vi "test_system_state-machine.vi"() -> ()   [LabVIEW 2019]
uses:
  Ctrl/main_system.ctl
panel:
  in  "정지":bool
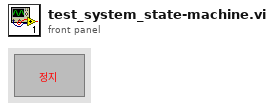
[diagram p1: front panel]
types:
  T1 = typedef "main_system.ctl" = enum16{"init state", "start point check", "end point check", "start angle check", "stop", "wait", "waypoint check"}
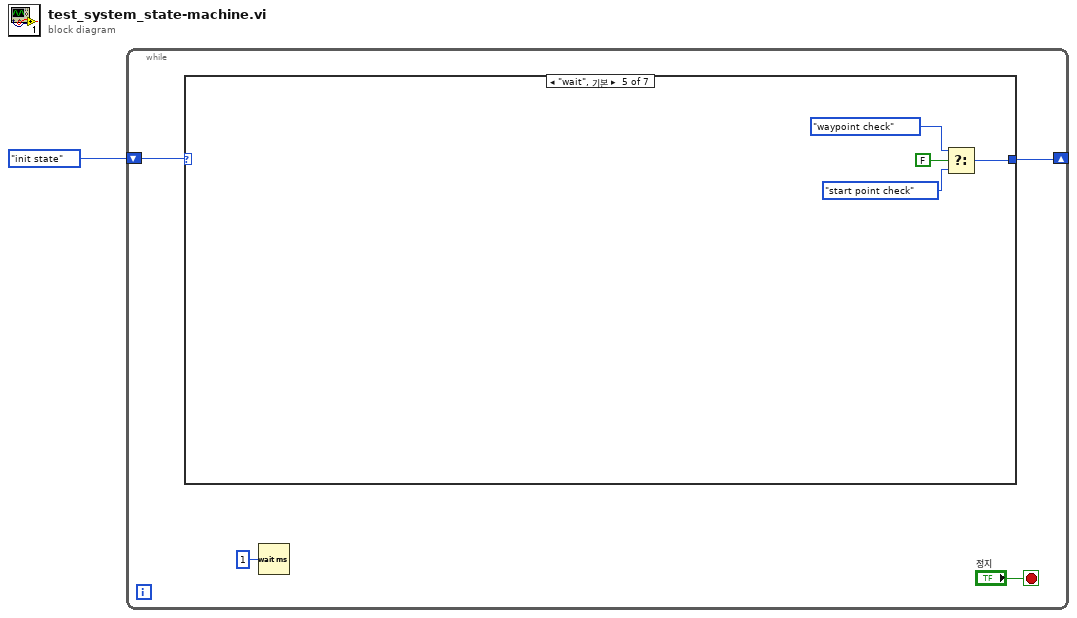
[diagram p0: block diagram]
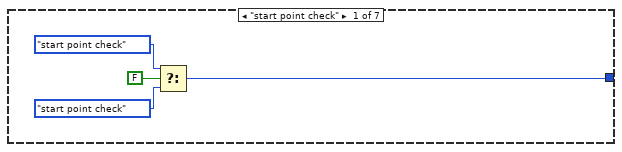
[diagram p2: hidden frame]
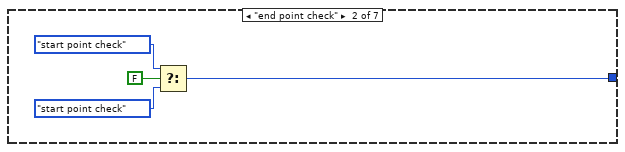
[diagram p3: hidden frame]
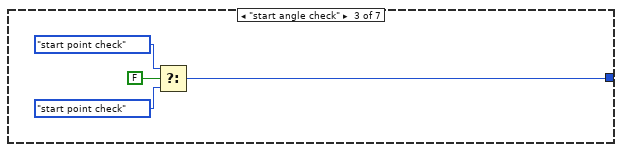
[diagram p4: hidden frame]
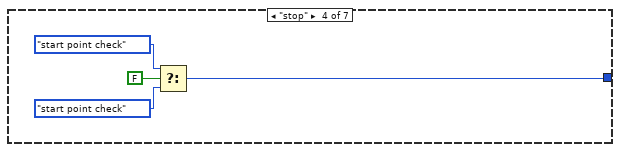
[diagram p5: hidden frame]
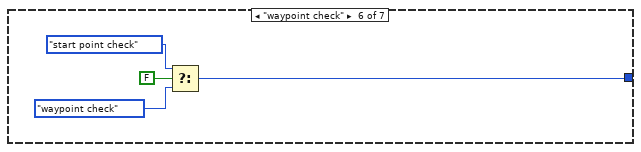
[diagram p6: hidden frame]
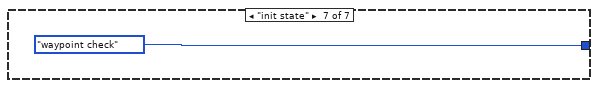
[diagram p7: hidden frame]
diagram:
  n1 = while {
    shift-right: [w2] -> _
    shift-left: main_system."init state" ("cmd") -> [w3]
    stop <- "정지" stop-if-true
    n2 = case shown="\"wait\", 기본" w3 {
      tunnel: [w9 w10 w14 w18 w22 w26 main_system."waypoint check" ("cmd")] -> w2
      frame "start point check" {
        n3 = Select(t=main_system."start point check" ("cmd"), s=FALSE, f=main_system."start point check" ("cmd")) -> (s? t:f=w9:T1)
      }
      frame "end point check" {
        n4 = Select(t=main_system."start point check" ("cmd"), s=FALSE, f=main_system."start point check" ("cmd")) -> (s? t:f=w10:T1)
      }
      frame "start angle check" {
        n5 = Select(t=main_system."start point check" ("cmd"), s=FALSE, f=main_system."start point check" ("cmd")) -> (s? t:f=w14:T1)
      }
      frame "stop" {
        n6 = Select(t=main_system."start point check" ("cmd"), s=FALSE, f=main_system."start point check" ("cmd")) -> (s? t:f=w18:T1)
      }
      frame "wait", Default {
        n7 = Select(t=main_system."waypoint check" ("cmd"), s=FALSE, f=main_system."start point check" ("cmd")) -> (s? t:f=w22:T1)
      }
      frame "waypoint check" {
        n8 = Select(t=main_system."start point check" ("cmd"), s=FALSE, f=main_system."waypoint check" ("cmd")) -> (s? t:f=w26:T1)
      }
      frame "init state" {
      }
    }
    n9 = Wait (ms)(milliseconds to wait=u32 1 ("대기 시간 (ms)")) -> ()  [unwired: 1 out]
  }
